vi "CRYExport data to tab-delimited.vi"(2 "Data/Wave(if true=wave)?":bool, 4 "Comment":string, 5 "File exists & overwrite (F)":bool, 6 "Format info":T1, 7 "Use format info? (F)":bool, 8 "suppress file output (false)":bool, 9 "indices to save (not wired: all)":i16[](array[numeric]), 10 "data series":string[](array[string]), 11 "File path (not wired: dialogue)":path) -> (0 "error/cancelled?":bool, 1 "tab-delimited output string":string, 3 "File path out":path)   [LabVIEW 2013]
uses:
  Data/CRYData & result stacks global.vi
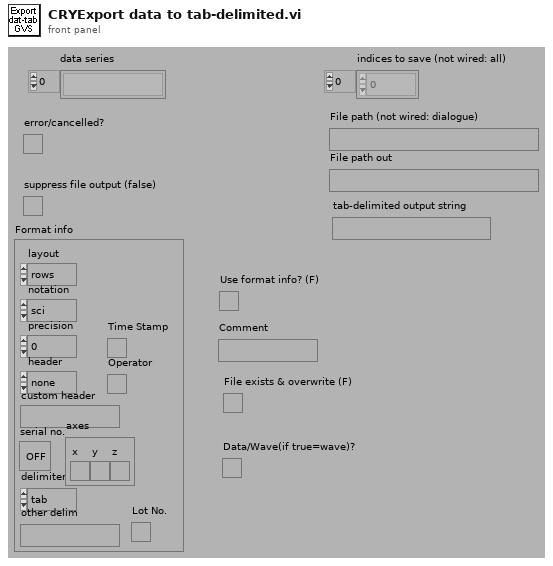
[diagram p1: front panel]
types:
  T1 = cluster{"layout":enum16{"rows", "columns"}, "notation":enum16{"sci", "float"}, "precision":i32, "header":enum16{"none", "standard", "custom"}, "custom header":string, "serial no.":bool, "delimiter":enum16{"tab", "comma", "space", "other"}, "other delim":string, "axes":cluster{"x":bool, "y":bool, "z":bool}, "Lot No.":bool, "Operator":bool, "Time Stamp":bool}
  T2 = enum16{"open", "open or create", "create or replace", "create"}
  T3 = enum16{"read/write", "read-only", "write-only", "write-only (truncate)"}
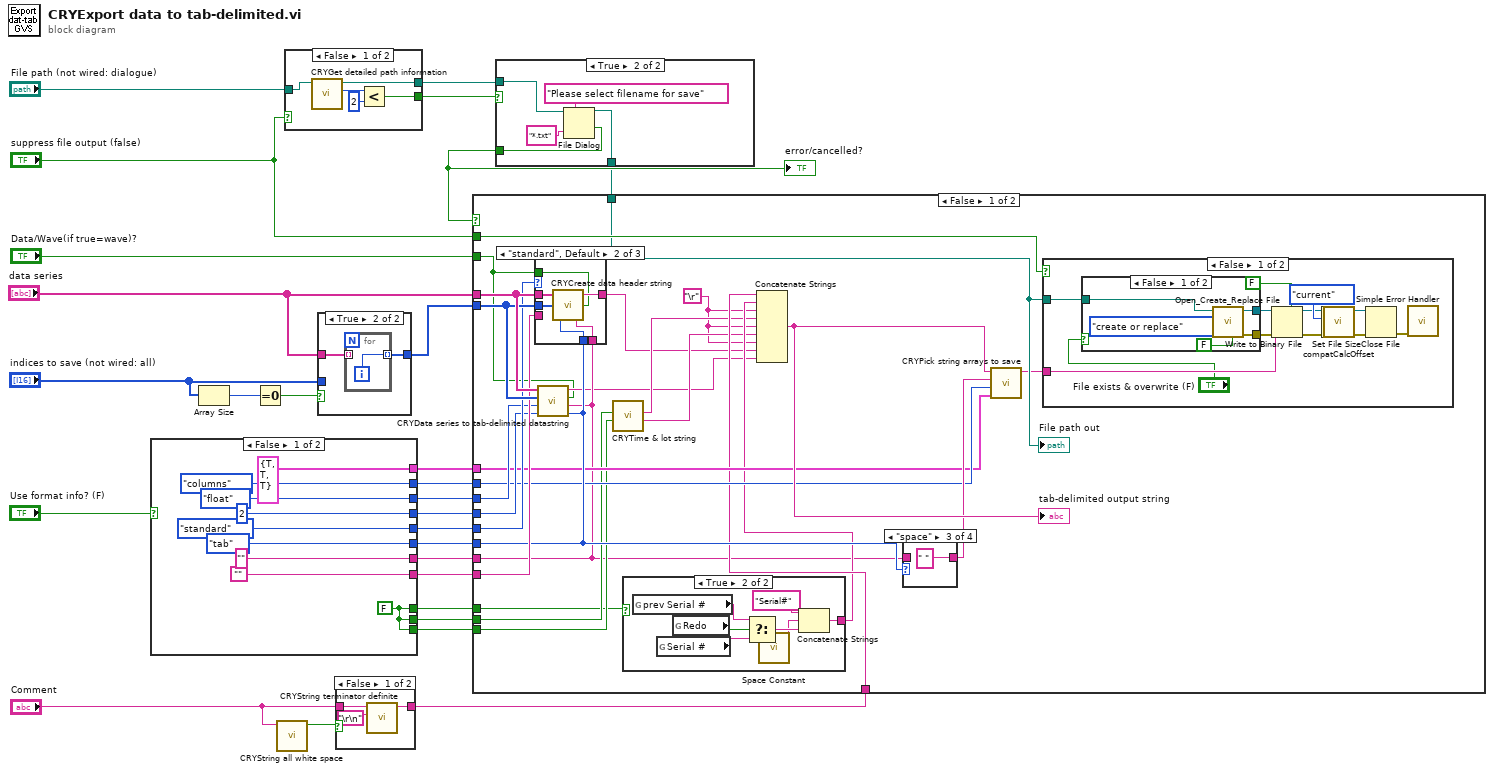
[diagram p0: block diagram]
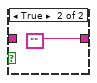
[diagram p2: hidden frame]
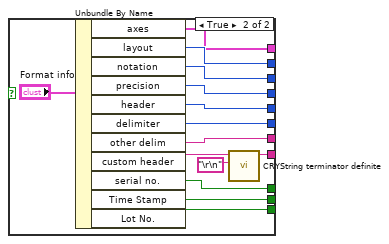
[diagram p3: hidden frame]
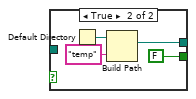
[diagram p4: hidden frame]
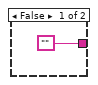
[diagram p5: hidden frame]
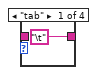
[diagram p6: hidden frame]
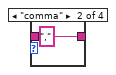
[diagram p7: hidden frame]
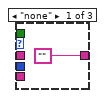
[diagram p9: hidden frame]
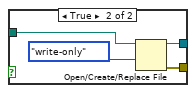
[diagram p11: hidden frame]
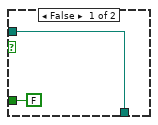
[diagram p14: hidden frame]
diagram:
  n1 = case shown="False" "Use format info? (F)" {
    tunnel: [enum16{"none", "standard", "custom"}."standard" ("header") w49] -> w16
    tunnel: ["" w45] -> w15
    tunnel: [enum16{"rows", "columns"}."columns" ("layout") w48] -> w14
    tunnel: [2 ("precision") w47] -> w13
    tunnel: [enum16{"sci", "float"}."float" ("notation") w46] -> w12
    tunnel: [enum16{"tab", "comma", "space", "other"}."tab" ("delimiter") w42] -> w10
    tunnel: ["" ("other delim") w41] -> w9
    tunnel: [cluster{"x":bool, "y":bool, "z":bool} {"x"=TRUE, "y"=TRUE, "z"=TRUE} ("axes") w40] -> w6
    tunnel: [w28 w39] -> w3
    tunnel: [w28 w38] -> w5
    tunnel: [w28 w37] -> w4
    frame False {
      w28 = FALSE ("serial no.")
    }
    frame True {
      n2 = Unbundle By Name("Format info") -> ("axes"=w40:cluster{"x":bool, "y":bool, "z":bool}, "layout"=w48:enum16{"rows", "columns"}, "notation"=w46:enum16{"sci", "float"}, "precision"=w47:i32, "header"=w49:enum16{"none", "standard", "custom"}, "delimiter"=w42:enum16{"tab", "comma", "space", "other"}, "other delim"=w41:string, "custom header"=w44:string, "serial no."=w39:bool, "Time Stamp"=w38:bool, "Lot No."=w37:bool)
      n3 = call "CRYString terminator definite.vi"("Terminator"="\r\n", "String in"=w44) -> ("String out"=w45:string)  [unwired: 9 in]
    }
  }
  n4 = Array Size(array="indices to save (not wired: all)") -> (size(s)=w26:i32)
  n5 = Equal To 0?(x=w26) -> (x = 0?=w27:bool)
  n6 = call "CRYString all white space.vi"("String"="Comment") -> ("Nothing but white space?"=w7:bool)  [unwired: 10 in]
  n7 = case shown="False" "suppress file output (false)" {
    tunnel: "File path (not wired: dialogue)" -> [w55 _]
    tunnel: [w54 w57] -> w24
    tunnel: [w51 FALSE] -> w25
    frame False {
      n8 = call "CRYGet detailed path information.vi"("complete path"=w55) -> ("portion type"=w53:i16, "longest valid portion"=w54:path)  [unwired: 9 in]
      n9 = Less?(x=w53, y=i16 2) -> (x < y?=w51:bool)
    }
    frame True {
      n10 = Default Directory() -> (w59:path)
      n11 = Build Path(base path=w59, name or relative path="temp") -> (appended path=w57:path)
    }
  }
  n12 = case shown="True" w27 {
    tunnel: "data series" -> [_ w62]
    tunnel: "indices to save (not wired: all)" -> [w60 _]
    tunnel: [w60 w61] -> w20
    frame False {
    }
    frame True {
      n13 = for {
        tunnel: [w63] -> w61 mode=indexing
        tunnel: w62 -> [_] mode=indexing
        i -> [w63]
      }
    }
  }
  n14 = case shown="False" w7 {
    tunnel: "Comment" -> [w66 _]
    tunnel: [w64 ""] -> w11
    frame False {
      n15 = call "CRYString terminator definite.vi"("Terminator"="\r\n", "String in"=w66) -> ("String out"=w64:string)  [unwired: 9 in]
    }
    frame True {
    }
  }
  n16 = case shown="True" w25 {
    tunnel: [FALSE w71] -> w21
    tunnel: w24 -> [w69 w70]
    tunnel: [w69 w73] -> w19
    frame False {
    }
    frame True {
      n17 = File Dialog(6:"*.txt" ("pattern"), 7:"Please select filename for save" ("prompt"), 11:w70) -> (1:w71:bool, 3:w73:path)  [unwired: 1 in, 5 out]
    }
  }
  "error/cancelled?" <- w21
  n18 = case shown="False" w21 {
    tunnel: "data series" -> [w100 _]
    tunnel: w20 -> [w99 _]
    tunnel: w19 -> [w93 _]
    tunnel: "suppress file output (false)" -> [w98 _]
    tunnel: w16 -> [w97 _]
    tunnel: w15 -> [w96 _]
    tunnel: w14 -> [w88 _]
    tunnel: w13 -> [w95 _]
    tunnel: w12 -> [w94 _]
    tunnel: w11 -> [w86 _]
    tunnel: w10 -> [w92 _]
    tunnel: w9 -> [w77 _]
    tunnel: w6 -> [w87 _]
    tunnel: w5 -> [w85 _]
    tunnel: w4 -> [w84 _]
    tunnel: w3 -> [w83 _]
    tunnel: "Data/Wave(if true=wave)?" -> [w75 _]
    frame False {
      w79 = "\r"
      n19 = case shown="\"standard\", Default" w97 {
        tunnel: w100 -> [_ w119 _]
        tunnel: w99 -> [_ w118 _]
        tunnel: ["" w117 w120] -> w78
        tunnel: w96 -> [_ _ w120]
        tunnel: w77 -> [_ w116 _]
        tunnel: w92 -> [_ w115 _]
        tunnel: w75 -> [_ w114 _]
        frame "none" {
        }
        frame "standard", Default {
          n20 = call "CRYCreate data header string.vi"("other delim"=w116, "Data/Wave(if true=wave)?"=w114, "delimiter"=w115, "indices to save"=w118, "data series"=w119) -> ("export file header"=w117:string)
        }
        frame "custom" {
        }
      }
      n21 = call "CRYData series to tab-delimited datastring.vi"("delimiter"=w92, "other delim"=w77, "Data/Wave(if true=wave)?"=w75, "precision"=w95, "notation"=w94, "indices to save"=w99, "data series"=w100) -> ("tab-delimited data string"=w76:string)
      n22 = call "CRYTime & lot string.vi"("Lot No."=w84, "Time Stamp"=w85) -> ("Lot string"=w80:string, "Time string"=w81:string)  [unwired: 6 in, 2 out]
      n23 = case shown="True" w83 {
        tunnel: ["" w102] -> w82
        frame False {
        }
        frame True {
          n24 = global read "CRYData & result stacks global.vi" "prev Serial #"() -> (w107:string)
          n25 = global read "CRYData & result stacks global.vi" "Serial #"() -> (w108:string)
          n26 = global read "CRYData & result stacks global.vi" "Redo"() -> (w106:bool)
          n27 = Select(t=w107, s=w106, f=w108) -> (s? t:f=w105:string)
          n28 = call <vilib>:"Space Constant.vi"() -> ("String"=w103:string)
          n29 = Concatenate Strings("Serial#" ("string"), w103, w105) -> (w102:string)
        }
      }
      n30 = Concatenate Strings(w86, w82, w79, w81, w79, w80, w79, w78, w76) -> (w90:string)
      "tab-delimited output string" <- w90
      n31 = case shown="\"space\"" w92 {
        tunnel: w77 -> [_ _ _ w112]
        tunnel: ["\t" "," " " w112] -> w89
        frame "tab" {
        }
        frame "comma" {
        }
        frame "space" {
        }
        frame Default {
        }
      }
      n32 = call "CRYPick string arrays to save.vi"("Axes"=w87, "Layout"=w88, "Delimiter"=w89, "Spreadsheet string"=w90) -> ("Spreadsheet string out"=w91:string)  [unwired: 7 in]
      n33 = case shown="False" w98 {
        tunnel: w91 -> [w127 _]
        tunnel: w93 -> [w126 _]
        frame False {
          n34 = case shown="False" "File exists & overwrite (F)" {
            tunnel: w126 -> [w139 w142]
            tunnel: [w138 w144] -> w135
            tunnel: [w137 w143] -> w134
            frame False {
              n35 = call <vilib>:"Open_Create_Replace File.vi"("advisory dialog? (display:T)"=FALSE, "function (open:0)"=T2."create or replace", "file path"=w139) -> ("error out"=w137:errorcluster, "refnum"=w138:refnum<file>)  [unwired: 4 in, 3 out]
            }
            frame True {
              n36 = Open/Create/Replace File(file path (use dialog)=w142, access (0:read/write)=T3."write-only" ("open mode (0)")) -> (refnum out=w144:refnum<file>, error out=w143:errorcluster)  [unwired: 1 in, 4 out]
            }
          }
          n37 = Write to Binary File(file (use dialog)=w135, data=w127, error in=w134, 5:FALSE ("预置数组或字符串大小？(T)")) -> (refnum out=w131:refnum<file>, error out=w132:errorcluster)  [unwired: 3 out]
          n38 = call <vilib>:"compatCalcOffset.vi"("error in"=w132, "pos mode (0:1)"=enum16{"start", "end", "current"}."current", "refnum"=w131) -> ("error out"=w123:errorcluster, "offset"=w122:i32, "dup refnum"=w121:refnum<file>)  [unwired: 1 in, 5 out]
          n39 = Set File Size(4:w123, 6:w122, 7:w121) -> (0:w129:errorcluster, 3:w130:refnum<file>)
          n40 = Close File(refnum=w130, error in=w129) -> (error out=w128:errorcluster)  [unwired: 1 out]
          n41 = call <vilib>:"Simple Error Handler.vi"("error in (no error)"=w128) -> ()  [unwired: 1 in, 8 out]
        }
        frame True {
        }
      }
      "File path out" <- w93
    }
    frame True {
    }
  }
